vi "Temperature_Converter.vi"() -> ()   [LabVIEW 2019]
panel:
  in  "To: Unit":enum16{"F", "C", "K"}(ring)
  in  "From: Unit":enum16{"F", "C", "K"}(ring)
  in  "Exit Button":bool
  in  "Convert Button":bool
  out "Your Result":dbl
  in  "Input a value":i32
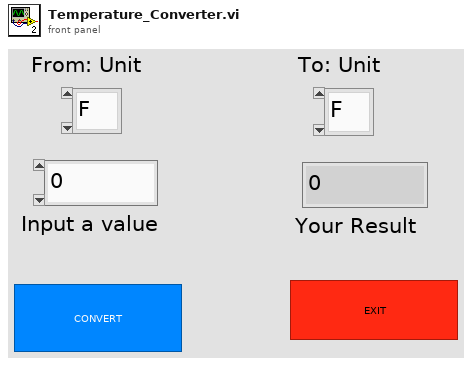
[diagram p1: front panel]
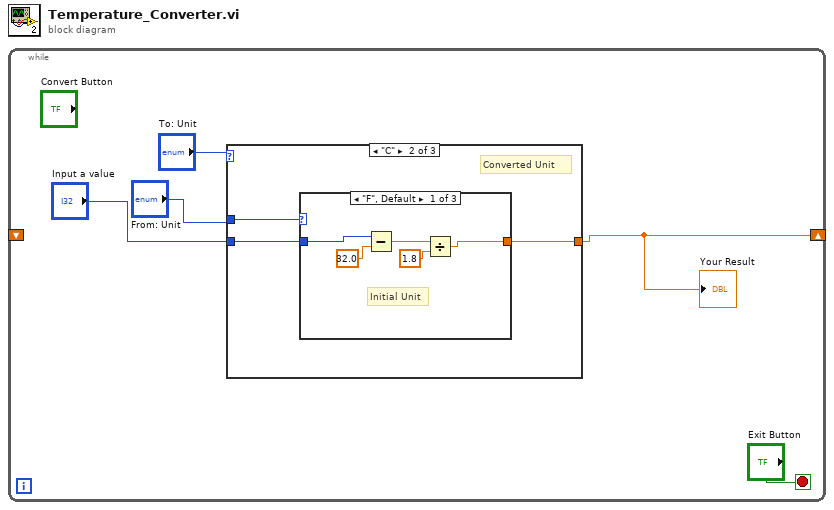
[diagram p0: block diagram]
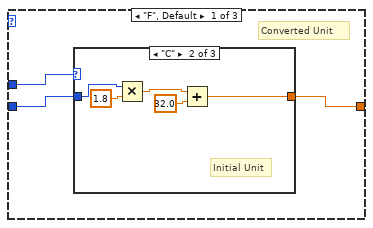
[diagram p2: hidden frame]
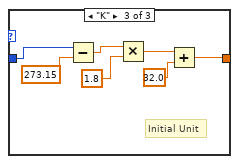
[diagram p4: hidden frame]
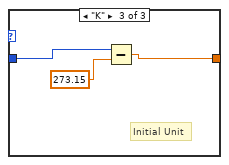
[diagram p6: hidden frame]
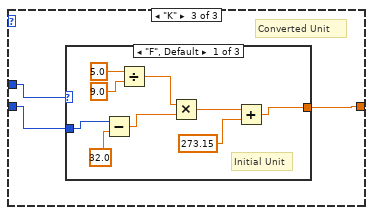
[diagram p7: hidden frame]
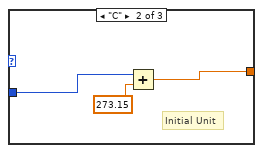
[diagram p8: hidden frame]
diagram:
  n1 = while {
    shift-right: [w2] -> _
    shift-left: _ -> [_]
    stop <- "Exit Button" stop-if-true
    n2 = case shown="\"C\"" "To: Unit" {
      tunnel: "From: Unit" -> [w8 w24 w36]
      tunnel: "Input a value" -> [w7 w23 w35]
      tunnel: [w6 w22 w34] -> w2
      frame "F", Default {
        # "Converted Unit"
        n3 = case shown="\"C\"" w8 {
          tunnel: w7 -> [w9 w11 w20]
          tunnel: [w9 w10 w17] -> w6
          frame "F", Default {
            # "Same Unit so no change"
            # "Initial Unit"
          }
          frame "C" {
            # "Initial Unit"
            n4 = Multiply(x=w11, y=1.8) -> (x*y=w12:dbl)
            n5 = Add(x=w12, y=32.0) -> (x+y=w10:dbl)
          }
          frame "K" {
            # "Initial Unit"
            n6 = Subtract(x=w20, y=273.15) -> (x-y=w18:dbl)
            n7 = Multiply(x=w18, y=1.8) -> (x*y=w15:dbl)
            n8 = Add(x=w15, y=32.0) -> (x+y=w17:dbl)
          }
        }
      }
      frame "C" {
        # "Converted Unit"
        n9 = case shown="\"F\", Default" w24 {
          tunnel: w23 -> [w25 w30 w32]
          tunnel: [w29 w30 w31] -> w22
          frame "F", Default {
            # "Initial Unit"
            n10 = Subtract(x=w25, y=32.0) -> (x-y=w27:dbl)
            n11 = Divide(x=w27, y=1.8) -> (x/y=w29:dbl)
          }
          frame "C" {
            # "Same Unit so no change"
            # "Initial Unit"
          }
          frame "K" {
            # "Initial Unit"
            n12 = Subtract(x=w32, y=273.15) -> (x-y=w31:dbl)
          }
        }
      }
      frame "K" {
        # "Converted Unit"
        n13 = case shown="\"F\", Default" w36 {
          tunnel: w35 -> [w44 w47 w49]
          tunnel: [w37 w46 w49] -> w34
          frame "F", Default {
            # "Initial Unit"
            n14 = Subtract(x=w44, y=32.0) -> (x-y=w40:dbl)
            n15 = Divide(x=5.0, y=9.0) -> (x/y=w41:dbl)
            n16 = Multiply(x=w41, y=w40) -> (x*y=w39:dbl)
            n17 = Add(x=w39, y=273.15) -> (x+y=w37:dbl)
          }
          frame "C" {
            # "Initial Unit"
            n18 = Add(x=w47, y=273.15) -> (x+y=w46:dbl)
          }
          frame "K" {
            # "Same Unit so no change"
            # "Initial Unit"
          }
        }
      }
    }
    "Your Result" <- w2
  }
